vi "Get Number VS Speeds.vi"(8 "error in (no error)":errorcluster, 11 "speeds":i32) -> (0 "error out":errorcluster, 2 "function return":u32, 3 "speeds out":i32)   [LabVIEW 2014, in "atmcd32d.lvlib"]
doc: "unsigned int WINAPI GetNumberVSSpeeds(int * speeds);"
uses:
  atmcd32d.lvlib
  atmcd32d.dll
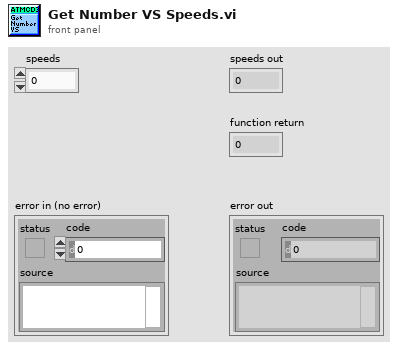
[diagram p1: front panel]
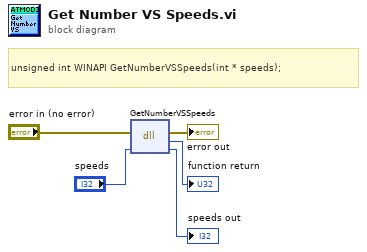
[diagram p0: block diagram]
diagram:
  # "unsigned int WINAPI GetNumberVSSpeeds(int * speeds);"
  n1 = dll-call lib="C:/Users/Bakir/Documents/Lambda2-Testing/lib/Andorlib/atmcd32d.*" fn="GetNumberVSSpeeds"(error in="error in (no error)", "speeds"="speeds") -> (error out=→"error out":errorcluster, →"function return":u32, "speeds"=→"speeds out":i32)  [unwired: 2 in, 1 out]
